vi "Parse-Find_Initial_Corner.vi"(11 "Color Array":u32[][](array[numeric])) -> (1 "Col Wall Thickness (px) (Y)":i32, 2 "Origin Y":i32, 4 "Wall Index Col":i32[](array[numeric]), 5 "Origin X":i32, 6 "Wall Index Row":i32[](array[numeric]), 7 "Row Wall Thickness (px) (X)":i32)   [LabVIEW 2020]
doc: "<B>Description:</B> Takes a 2D array of colors and scans it for the top corner and the wall thickness.\n\n<B>Date:</B> 1/2019\n<B>Author:</B> Luke Jarocki, Choose Movement Consulting, LLC"
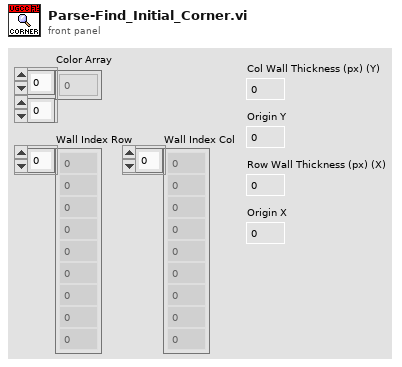
[diagram p1: front panel]
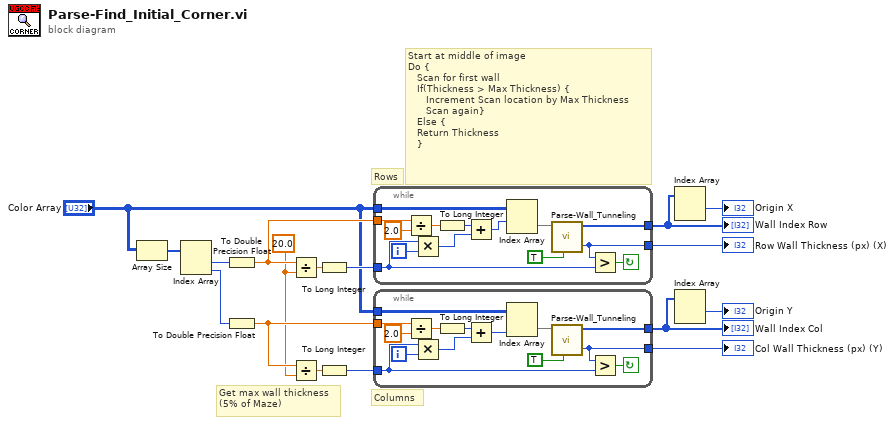
[diagram p0: block diagram]
diagram:
  w6 = 20.0 ("y")
  # "Start at middle of image\nDo {\n   Scan for first wall\n   If(Thickness > Max Thickness) {\n      Increment Scan location by Max Thickness\n      Scan again}\n   Else {\n   Return Thickness\n   }"
  # "Rows"
  # "Get max wall thickness\n(5% of Maze)"
  # "Columns"
  n1 = Array Size(array="Color Array") -> (size(s)=w17:i32[])
  n2 = Index Array(array=w17) -> (element #1=w16:i32, element #2=w11:i32)  [unwired: 2 in]
  n3 = To Double Precision Float(number=w16) -> (double precision float=w9:dbl)
  n4 = To Double Precision Float(number=w11) -> (double precision float=w10:dbl)
  n5 = Divide(x=w9, y=w6) -> (x/y=w15:dbl)
  n6 = Divide(x=w10, y=w6) -> (x/y=w8:dbl)
  n7 = To Long Integer(number=w15) -> (32bit integer=w14:i32)
  n8 = To Long Integer(number=w8) -> (32bit integer=w7:i32)
  n9 = while {
    tunnel: w14 -> [w23]
    tunnel: "Color Array" -> [w30]
    tunnel: w9 -> [w29]
    tunnel: [w19] -> w13
    tunnel: [w20] -> w5
    i -> [w24]
    stop <- w26 continue-if-true
    n10 = Divide(x=w29, y=2.0) -> (x/y=w27:dbl)
    n11 = Multiply(x=w23, y=w24) -> (x*y=w22:i32)
    n12 = To Long Integer(number=w27) -> (32bit integer=w21:i32)
    n13 = Add(x=w21, y=w22) -> (x+y=w25:i32)
    n14 = Index Array(array=w30, index (row)=w25) -> (element=w31:u32[])  [unwired: 1 in]
    n15 = call "Parse-Wall_Tunneling.vi"("Tunnal All (F)"=TRUE, "Line to Parse"=w31) -> ("Wall Center Index"=w20:i32[], "Wall Thickness (px)"=w19:i32)  [unwired: 6 in, 2 out]
    n16 = Greater?(x=w19, y=w23) -> (0:w26:bool)
  }
  "Row Wall Thickness (px) (X)" <- w13
  "Wall Index Row" <- w5
  n17 = while {
    tunnel: w7 -> [w38]
    tunnel: "Color Array" -> [w44]
    tunnel: w10 -> [w43]
    tunnel: [w33] -> w12
    tunnel: [w35] -> w4
    i -> [w39]
    stop <- w40 continue-if-true
    n18 = Divide(x=w43, y=2.0) -> (x/y=w41:dbl)
    n19 = Multiply(x=w38, y=w39) -> (x*y=w37:i32)
    n20 = To Long Integer(number=w41) -> (32bit integer=w36:i32)
    n21 = Add(x=w36, y=w37) -> (x+y=w34:i32)
    n22 = Index Array(array=w44, index (col)=w34) -> (element=w45:u32[])  [unwired: 1 in]
    n23 = call "Parse-Wall_Tunneling.vi"("Tunnal All (F)"=TRUE, "Line to Parse"=w45) -> ("Wall Center Index"=w35:i32[], "Wall Thickness (px)"=w33:i32)  [unwired: 6 in, 2 out]
    n24 = Greater?(x=w33, y=w38) -> (0:w40:bool)
  }
  "Wall Index Col" <- w4
  "Col Wall Thickness (px) (Y)" <- w12
  n25 = Index Array(array=w5) -> (element #1=→"Origin X":i32)  [unwired: 2 in, 1 out]
  n26 = Index Array(array=w4) -> (element #1=→"Origin Y":i32)  [unwired: 2 in, 1 out]
